vi "Decorator.vi"(10 "Actor":refnum<class "Actor.lvclass">, 11 "Decorator in":refnum<class "Decorator.lvclass">) -> (3 "Decorator out":refnum<class "Decorator.lvclass">)   [LabVIEW 2020, in "jettl.lvlib" / "Decorator.lvclass"]
uses:
  Decorator.lvclass
  Actor/Actor/Actor.lvclass
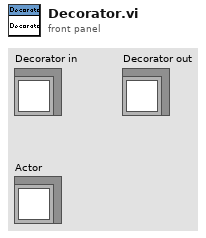
[diagram p1: front panel]
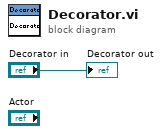
[diagram p0: block diagram]
diagram:
  "Decorator out" <- "Decorator in"
